vi "Spectra_cluster_to_f.E(f).vi"(1 "delta f":dbl format="%.2f", 2 "f":dbl format="%.2f", 3 "Spectra array":dbl[][](array[numeric]) format="%.2f") -> (0 "f.E(f) array":dbl[][](array[numeric]) format="%.2f")   [LabVIEW 2020]
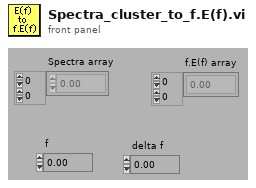
[diagram p1: front panel]
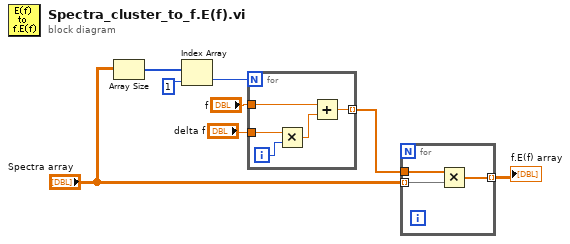
[diagram p0: block diagram]
diagram:
  n1 = Array Size(array="Spectra array") -> (size(s)=w4:i32[])
  n2 = Index Array(array=w4, index=1) -> (element=w5:i32)
  n3 = for {
    N: w5 -> [_]
    tunnel: "f" -> [w11]
    tunnel: "delta f" -> [w10]
    tunnel: [w9] -> w2 mode=indexing
    i -> [w13]
    n4 = Multiply(x=w10, y=w13) -> (x*y=w12:dbl)
    n5 = Add(x=w11, y=w12) -> (x+y=w9:dbl)
  }
  n6 = for {
    tunnel: "Spectra array" -> [w16] mode=indexing
    tunnel: w2 -> [w15]
    tunnel: [w14] -> w1 mode=indexing
    n7 = Multiply(x=w15, y=w16) -> (x*y=w14:dbl[])
  }
  "f.E(f) array" <- w1
